vi "Measurement UI.vi"() -> ()   [LabVIEW 2021, in "Gain And Offset_ADC.lvlib"]
uses:
  Gain And Offset_ADC.lvlib
panel:
  in  "MeasGraphs":enum32{"Transfer Function", "Hidden Controls"}(tab)
  out "TransferFunction":cluster{"Waveform":dbl[], "DMM readings":dbl[]}(graph) caption="FreqDomainGraph"
  in  "DMM resource name":string
  out "Offset":dbl
  out "Gain":dbl
  out "Channel name":string
  out "DMM readings":dbl[](array[numeric])
  out "ADC readings":dbl[](array[numeric])
  in  "Digital capture resource name":string
  in  "Analog source resource name":string
  out "MeasTable":string[][](table)
  in  "MeasSettingsOptions":i32(listbox)
  in  "DMM":string="DMM"
  in  "Digital capture":string="Digital capture"
  in  "Analog source":string="Analog source"
  in  "MeasSettings":bool
  in  "ADC parameters":string="ADC parameters"
  in  "DMM resolution":dbl(ring)=7.5 caption="RESOLUTION IN DIGITS" items=["3 1/2"=3.5, "4 1/2"=4.5, "5 1/2"=5.5, "6 1/2"=6.5, "7 1/2"=7.5]
  in  "DMM range":dbl=10.0 caption="RANGE" format="%#_6pV"
  in  "DMMResourceName":refnum<k15> caption="RESOURCE NAME"
  in  "Ramp stop":dbl=4.9 caption="RAMP STOP" format="%#_6pV"
  in  "Ramp start":dbl=-4.9 caption="RAMP START" format="%#_6pV"
  in  "Ramp samples":i32=10 caption="RAMP SAMPLES"
  in  "Analog source sample rate":dbl=1000.0 caption="SAMPLE RATE" format="%#_6pHz"
  in  "Digital capture samples":u32=10000 caption="NUMBER OF SAMPLES"
  in  "Input channel":i32 caption="INPUT CHANNEL" min=0 max=100 step=1
  in  "Full scale range":dbl=10.0 caption="FULL SCALE RANGE" format="%#_6pV"
  in  "Digital capture sample rate":dbl=800000.0 caption="SAMPLE RATE" format="%#_6pS/s"
  in  "DSGResourceName":tag caption="RESOURCE NAME"
  in  "DPIResourceName":refnum<k15> caption="RESOURCE NAME"
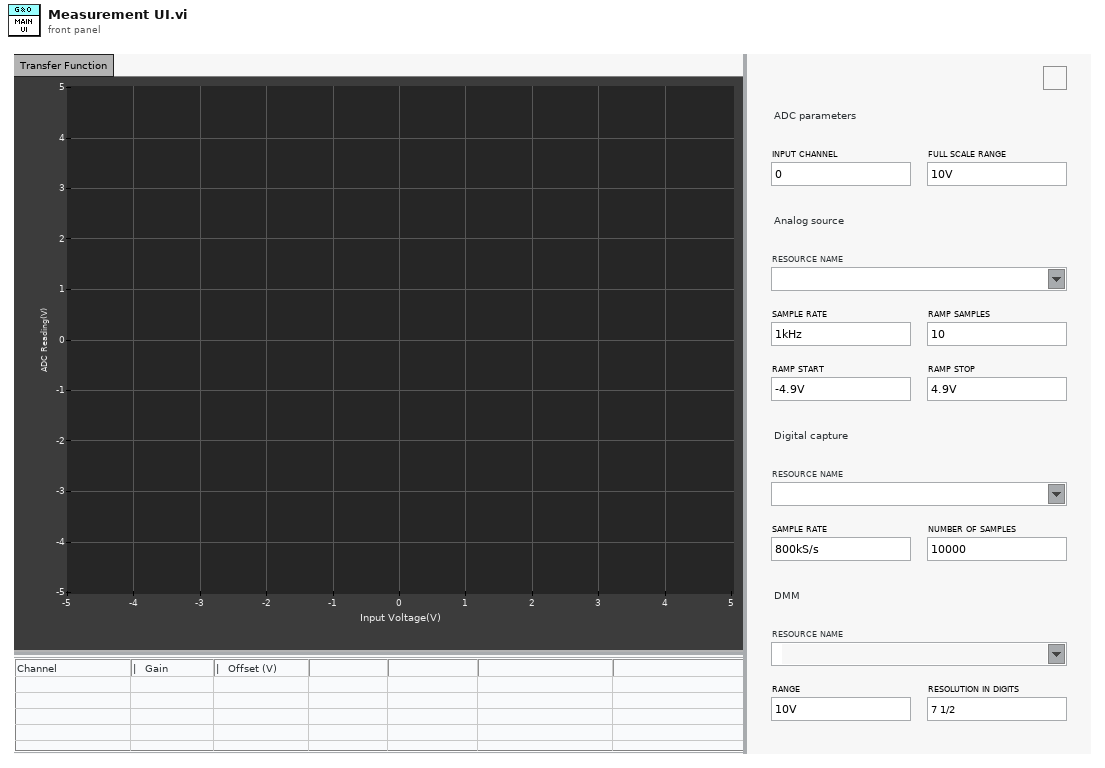
[diagram p1: front panel]
types:
  T1 = enum16{"open", "replace", "create", "open or create", "replace or create", "replace or create with confirmation"}
  T2 = cluster{"ADC readings":dbl[], "DMM readings":dbl[]}
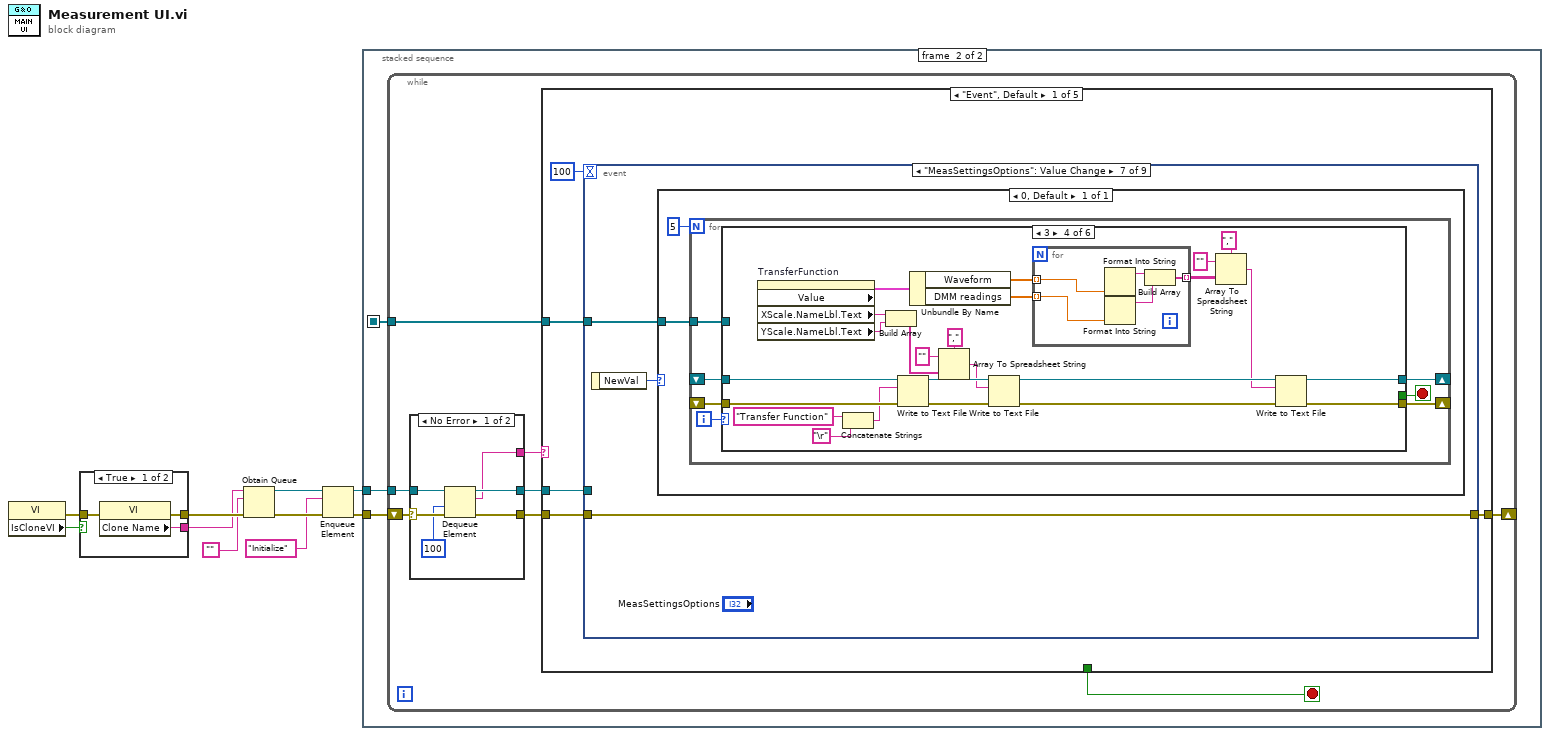
[diagram p0: block diagram]
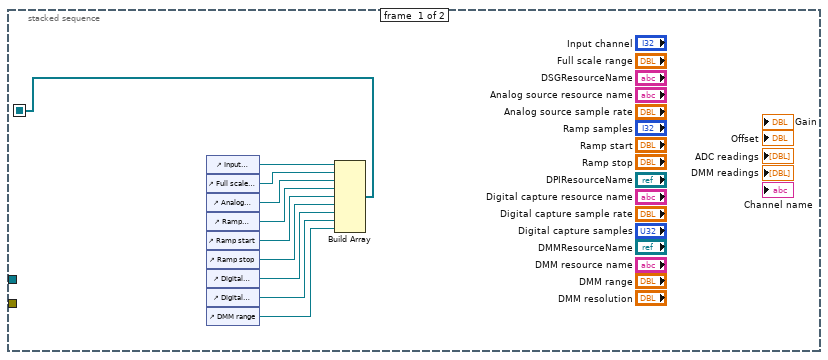
[diagram p2: hidden frame]
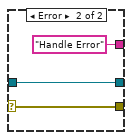
[diagram p3: hidden frame]
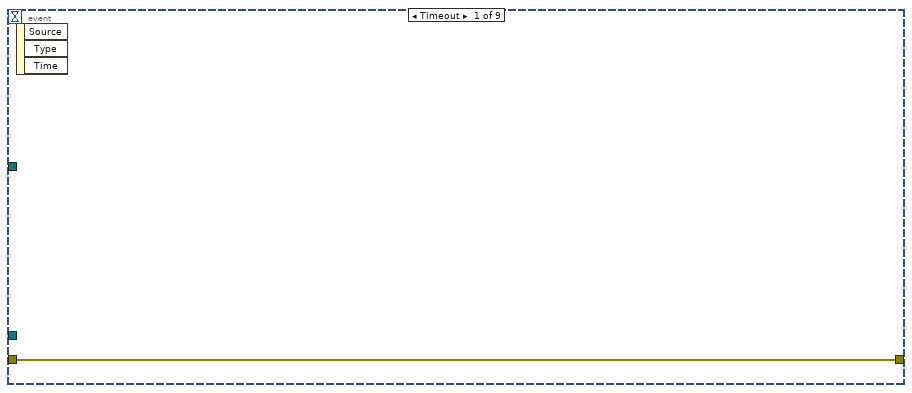
[diagram p4: hidden frame]
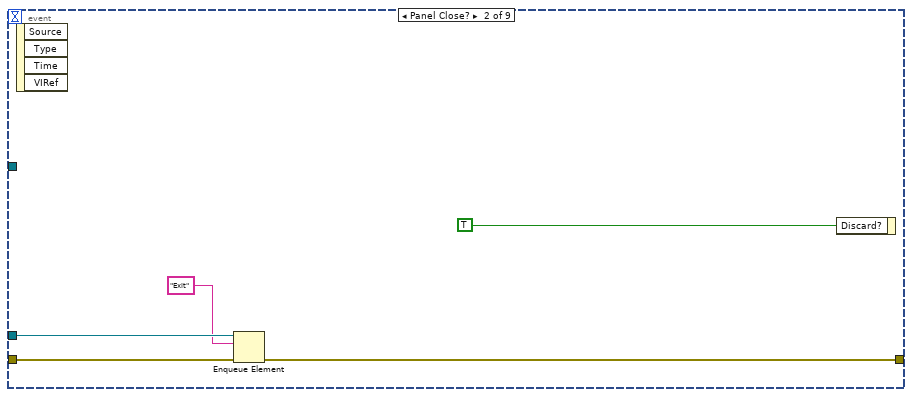
[diagram p5: hidden frame]
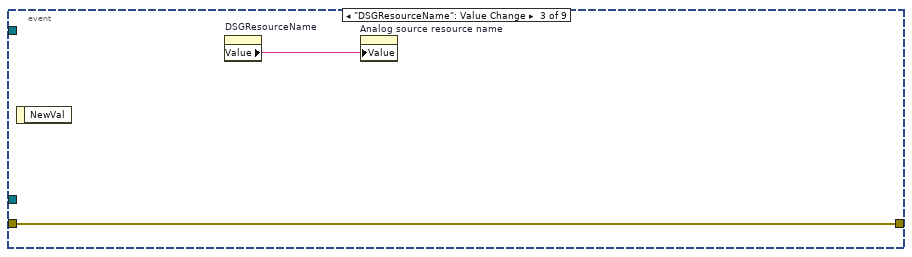
[diagram p6: hidden frame]
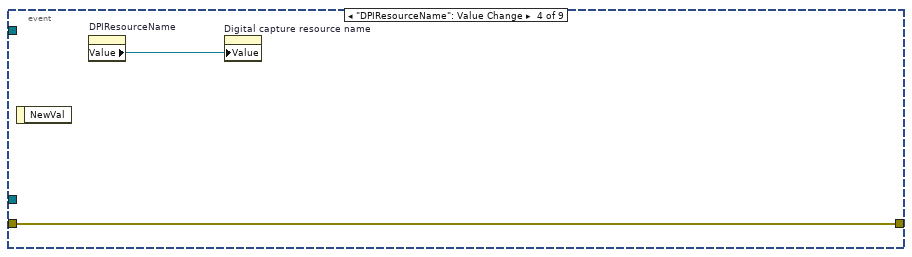
[diagram p7: hidden frame]
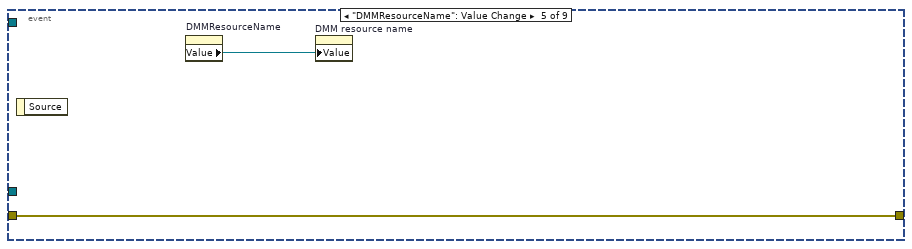
[diagram p8: hidden frame]
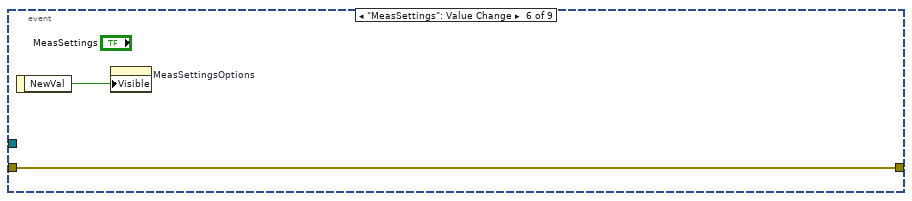
[diagram p9: hidden frame]
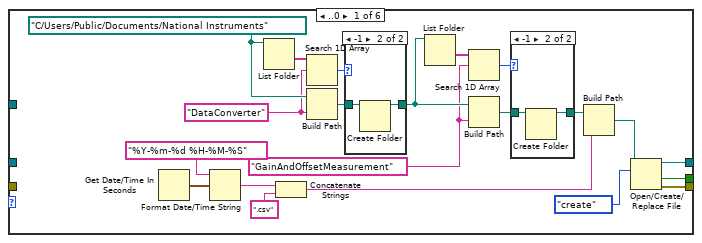
[diagram p10: hidden frame]
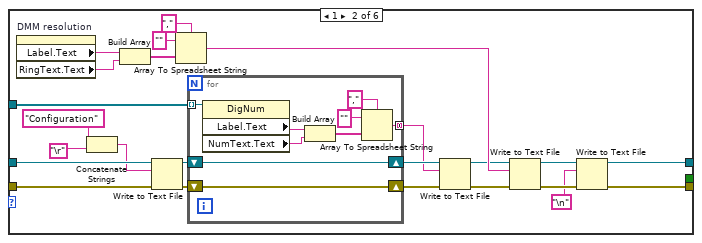
[diagram p13: hidden frame]
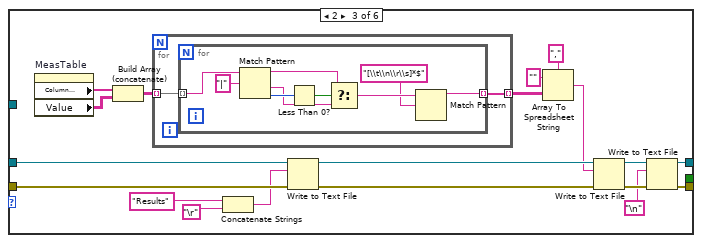
[diagram p14: hidden frame]
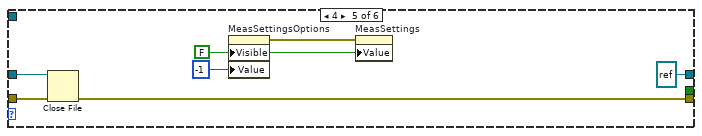
[diagram p15: hidden frame]
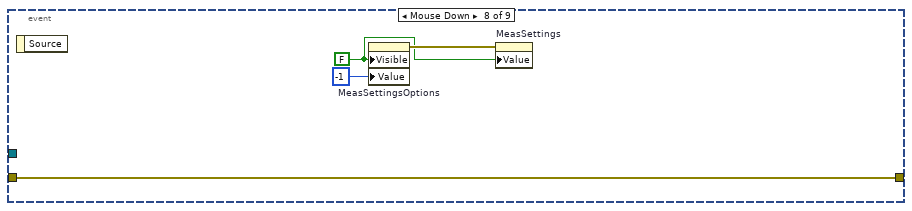
[diagram p17: hidden frame]
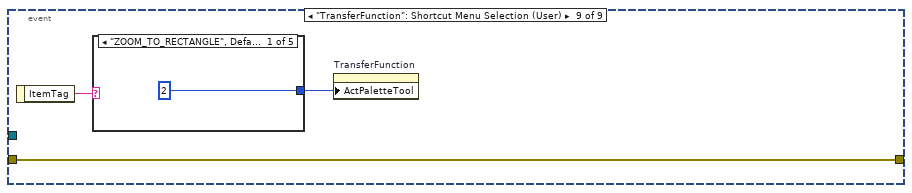
[diagram p18: hidden frame]
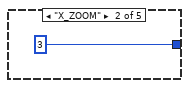
[diagram p19: hidden frame]
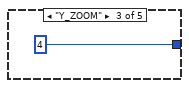
[diagram p20: hidden frame]
diagram:
  n1 = property class="VI"() -> (error out=w1:errorcluster, "IsCloneVI"=w2:bool)  [unwired: 2 in, 1 out]
  n2 = case shown="True" w2 {
    tunnel: [w13 w16] -> w10
    tunnel: [w12 w15] -> w9
    tunnel: w1 -> [w11 w14]
    frame True {
      n3 = property class="VI"(error in=w11) -> (error out=w13:errorcluster, "Clone Name"=w12:string)  [unwired: 1 in, 1 out]
    }
    frame False {
      n4 = property class="VI"(error in=w14) -> (error out=w16:errorcluster, "Name"=w15:string)  [unwired: 1 in, 1 out]
    }
  }
  n5 = Obtain Queue(name (unnamed)=w9, element data type="", error in (no error)=w10) -> (queue out=w6:refnum<queue>, error out=w8:errorcluster)  [unwired: 2 in, 1 out]
  n6 = Enqueue Element(queue=w6, element="Initialize", error in (no error)=w8) -> (queue out=w5:refnum<queue>, error out=w7:errorcluster)  [unwired: 1 in, 1 out]
  n7 = stacked-sequence {
    seq-local: [w17 _] -> [_ w27]
    tunnel: w7 -> [_ w29]
    tunnel: w5 -> [_ w28]
    frame #0 {
      n8 = control-ref of="Input channel"() -> (w26:refnum<vi>)
      n9 = control-ref of="Full scale range"() -> (w25:refnum<vi>)
      n10 = control-ref of="Analog source sample rate"() -> (w24:refnum<vi>)
      n11 = control-ref of="Ramp samples"() -> (w23:refnum<vi>)
      n12 = control-ref of="Ramp start"() -> (w22:refnum<vi>)
      n13 = control-ref of="Ramp stop"() -> (w21:refnum<vi>)
      n14 = control-ref of="Digital capture sample rate"() -> (w20:refnum<vi>)
      n15 = control-ref of="Digital capture samples"() -> (w19:refnum<vi>)
      n16 = control-ref of="DMM range"() -> (w18:refnum<vi>)
      n17 = Build Array(w26, w25, w24, w23, w22, w21, w20, w19, w18) -> (w17:refnum<vi>[])
    }
    frame #1 {
      n18 = while {
        shift-right: [w32] -> _
        shift-left: w29 -> [w37]
        tunnel: w28 -> [w35]
        tunnel: w27 -> [w30]
        stop <- w31 stop-if-true
        n19 = case shown="No Error" w37 {
          selector: w37 -> [w43 w46]
          tunnel: [w42 w46] -> w36
          tunnel: w35 -> [w41 w45]
          tunnel: [w40 w45] -> w34
          tunnel: [w39 "Handle Error"] -> w33
          frame No Error {
            n20 = Dequeue Element(queue=w41, timeout in ms (-1)=100, error in (no error)=w43) -> (queue out=w40:refnum<queue>, element=w39:string, error out=w42:errorcluster)  [unwired: 1 out]
          }
          frame Error {
          }
        }
        n21 = case shown="\"Event\", Default" w33 {
          tunnel: w36 -> [w50 w225 w239 w249 w250]
          tunnel: w34 -> [w48 _ _ w247 _]
          tunnel: [w51 w225 w239 w244 w250] -> w32
          tunnel: [_ FALSE _ TRUE _] -> w31
          tunnel: w30 -> [w47 _ _ _ _]
          frame "Event", Default {
            n22 = event shown="[6] \"MeasSettingsOptions\": Value Change" {
              selector: _ -> [_ _ _ _ _ _ _ _ _]
              dyn-events: _ -> [_ _ _ _ _ _ _ _ _]
              timeout: 100 -> [_ _ _ _ _ _ _ _ _]
              tunnel: [w52 w55 w59 w60 w62 w65 w68 w209 w210] -> w51
              tunnel: w50 -> [w52 w56 w59 w60 w62 w65 w68 w209 w210]
              tunnel: w48 -> [_ w54 _ _ _ _ _ _ _]
              tunnel: w47 -> [_ _ _ _ _ _ w66 _ _]
              event Timeout {
                n23 = event-data() -> ()  [unwired: 1 in, 3 out]
              }
              event Panel Close? {
                n24 = event-data() -> ()  [unwired: 1 in, 4 out]
                n25 = Enqueue Element(queue=w54, element="Exit", error in (no error)=w56) -> (error out=w55:errorcluster)  [unwired: 1 in, 2 out]
                n26 = event-data("Discard?"=TRUE) -> ()  [unwired: 1 in, 1 out]
              }
              event "DSGResourceName": Value Change {
                n27 = event-data() -> ()  [unwired: 1 in, 1 out]
                n28 = property on="DSGResourceName" class="DAQmxName"() -> ("Value"=w58:string)  [unwired: 2 in, 2 out]
                n29 = property on="Analog source resource name" class="Str"("Value"=w58) -> ()  [unwired: 2 in, 2 out]
              }
              event "DPIResourceName": Value Change {
                n30 = event-data() -> ()  [unwired: 1 in, 1 out]
                n31 = property on="DPIResourceName" class="IVIName"() -> ("Value"=w61:refnum<k15>)  [unwired: 2 in, 2 out]
                n32 = property on="Digital capture resource name" class="Str"("Value"=w61) -> ()  [unwired: 2 in, 2 out]
              }
              event "DMMResourceName": Value Change {
                n33 = event-data() -> ()  [unwired: 1 in, 1 out]
                n34 = property on="DMMResourceName" class="IVIName"() -> ("Value"=w63:refnum<k15>)  [unwired: 2 in, 2 out]
                n35 = property on="DMM resource name" class="Str"("Value"=w63) -> ()  [unwired: 2 in, 2 out]
              }
              event "MeasSettings": Value Change {
                n36 = event-data() -> ("NewVal"=w64:bool)  [unwired: 1 in]
                n37 = property on="MeasSettingsOptions" class="LstBox (strict)"("Visible"=w64) -> ()  [unwired: 2 in, 2 out]
              }
              event "MeasSettingsOptions": Value Change {
                n38 = event-data() -> ("NewVal"=w67:i32)  [unwired: 1 in]
                n39 = case shown="0, Default" w67 {
                  tunnel: w66 -> [w69]
                  frame 0, Default {
                    n40 = for {
                      N: 5 -> [_]
                      shift-right: [w75] -> _
                      shift-left: _ -> [w74]
                      shift-right: [w73] -> _
                      shift-left: _ -> [w72]
                      tunnel: w69 -> [w71]
                      i -> [w77]
                      stop <- w76 stop-if-true
                      n41 = case shown="3" w77 {
                        tunnel: [w91 _ _ _ _ _] -> w76
                        tunnel: [w97 w108 w143 w177 refnum<file> refnum ("refnum out") w205] -> w75
                        tunnel: w74 -> [_ w126 w156 w191 w200 w205]
                        tunnel: [w90 w106 w142 w176 w198 w204] -> w73
                        tunnel: w72 -> [_ w124 w155 w190 w199 w204]
                        tunnel: w71 -> [_ w128 _ _ _ _]
                        frame ..0 {
                          w86 = "GainAndOffsetMeasurement" ("prompt")
                          w93 = "DataConverter" ("prompt")
                          w96 = path "C:/Users/Public/Documents/National Instruments" ("base path")
                          n42 = Get Date/Time In Seconds() -> (seconds since 1Jan1904=w83:timestamp)
                          n43 = Format Date/Time String(time format string (%c)="%Y-%m-%d %H-%M-%S", seconds (now)=w83) -> (date/time string=w82:string)  [unwired: 1 in]
                          n44 = List Folder(path=w96) -> (folder names=w94:string[])  [unwired: 3 in, 3 out]
                          n45 = Concatenate Strings(w82, ".csv" ("string")) -> (w79:string)
                          n46 = Search 1D Array(1D array=w94, element=w93) -> (index of element=w92:i32)  [unwired: 1 in]
                          n47 = Build Path(base path=w96, name or relative path=w93) -> (appended path=w95:path)
                          n48 = case shown="-1" w92 {
                            tunnel: w95 -> [w102 w104]
                            tunnel: [w102 w103] -> w87
                            frame Default {
                            }
                            frame -1 {
                              n49 = Create Folder(path (use dialog)=w104) -> (created path=w103:path)  [unwired: 2 in, 2 out]
                            }
                          }
                          n50 = List Folder(path=w87) -> (folder names=w89:string[])  [unwired: 3 in, 3 out]
                          n51 = Search 1D Array(1D array=w89, element=w86) -> (index of element=w88:i32)  [unwired: 1 in]
                          n52 = Build Path(base path=w87, name or relative path=w86) -> (appended path=w85:path)
                          n53 = case shown="-1" w88 {
                            tunnel: w85 -> [w99 w101]
                            tunnel: [w99 w100] -> w80
                            frame Default {
                            }
                            frame -1 {
                              n54 = Create Folder(path (use dialog)=w101) -> (created path=w100:path)  [unwired: 2 in, 2 out]
                            }
                          }
                          n55 = Build Path(base path=w80, name or relative path=w79) -> (appended path=w78:path)
                          n56 = Open/Create/Replace File(file path (use dialog)=w78, operation (0:open)=T1."create") -> (refnum out=w97:refnum<file>, cancelled=w91:bool, error out=w90:errorcluster)  [unwired: 4 in]
                        }
                        frame 1 {
                          n57 = property on="DMM resolution" class="Ring (strict)"() -> ("Label.Text"=w120:string, "RingText.Text"=w119:string)  [unwired: 2 in, 2 out]
                          n58 = Concatenate Strings("Configuration" ("format string"), "\r") -> (w121:string)
                          n59 = Build Array(w120, w119) -> (w116:string[])
                          n60 = Write to Text File(file (use dialog)=w126, text=w121, error in=w124) -> (refnum out=w127:refnum<file>, error out=w125:errorcluster)  [unwired: 1 in, 1 out]
                          n61 = Array To Spreadsheet String(delimiter (Tab)=",", array=w116, 3:"" ("format string")) -> (spreadsheet string=w115:string)
                          n62 = for {
                            tunnel: w128 -> [w137] mode=indexing
                            shift-right: [w134] -> w114
                            shift-left: w127 -> [w134]
                            shift-right: [w133] -> w112
                            shift-left: w125 -> [w133]
                            tunnel: [w129] -> w110 mode=concatenating
                            n63 = property class="DigNum"(reference=w137) -> ("Label.Text"=w136:string, "NumText.Text"=w135:string)  [unwired: 1 in, 2 out]
                            n64 = Build Array(w136, w135) -> (w130:string[])
                            n65 = Array To Spreadsheet String(delimiter (Tab)=",", array=w130, 3:"" ("format string")) -> (spreadsheet string=w129:string)
                          }
                          n66 = Write to Text File(file (use dialog)=w114, text=w110, error in=w112) -> (refnum out=w113:refnum<file>, error out=w111:errorcluster)  [unwired: 1 in, 1 out]
                          n67 = Write to Text File(file (use dialog)=w113, text=w115, error in=w111) -> (refnum out=w109:refnum<file>, error out=w107:errorcluster)  [unwired: 1 in, 1 out]
                          n68 = Write to Text File(file (use dialog)=w109, text="\n", error in=w107) -> (refnum out=w108:refnum<file>, error out=w106:errorcluster)  [unwired: 1 in, 1 out]
                        }
                        frame 2 {
                          n69 = property on="MeasTable" class="Tbl (strict)"() -> ("Column Headers[]"=w153:string[], "Value"=w152:string[][])  [unwired: 2 in, 2 out]
                          n70 = Build Array (concatenate)(w153, w152) -> (w151:string[][])
                          n71 = for {
                            tunnel: w151 -> [w158] mode=indexing
                            tunnel: [w157] -> w150 mode=indexing
                            n72 = for {
                              tunnel: w158 -> [w160] mode=indexing
                              tunnel: [w159] -> w157 mode=indexing
                              n73 = Match Pattern(string=w160, regular expression="|") -> (before substring=w164:string, after substring=w163:string, offset past match=w166:i32)  [unwired: 1 in, 1 out]
                              n74 = Less Than 0?(x=w166) -> (x < 0?=w165:bool)
                              n75 = Select(t=w164, s=w165, f=w163) -> (s? t:f=w162:string)
                              n76 = Match Pattern(string=w162, regular expression="[\\t\\n\\r\\s]*$") -> (before substring=w159:string)  [unwired: 1 in, 3 out]
                            }
                          }
                          n77 = Concatenate Strings("Results" ("element"), "\r") -> (w138:string)
                          n78 = Write to Text File(file (use dialog)=w156, text=w138, error in=w155) -> (refnum out=w154:refnum<file>, error out=w146:errorcluster)  [unwired: 1 in, 1 out]
                          n79 = Array To Spreadsheet String(delimiter (Tab)=",", array=w150, 3:"" ("format string")) -> (spreadsheet string=w147:string)
                          n80 = Write to Text File(file (use dialog)=w154, text=w147, error in=w146) -> (refnum out=w145:refnum<file>, error out=w144:errorcluster)  [unwired: 1 in, 1 out]
                          n81 = Write to Text File(file (use dialog)=w145, text="\n", error in=w144) -> (refnum out=w143:refnum<file>, error out=w142:errorcluster)  [unwired: 1 in, 1 out]
                        }
                        frame 3 {
                          n82 = property on="TransferFunction" class="XYGraph (strict)"() -> ("Value"=w170:cluster{"Waveform":dbl[], "DMM readings":dbl[]}, "XScale.NameLbl.Text"=w187:string, "YScale.NameLbl.Text"=w186:string)  [unwired: 2 in, 2 out]
                          n83 = Concatenate Strings("Transfer Function" ("string"), "\r") -> (w188:string)
                          n84 = Build Array(w187, w186) -> (w185:string[])
                          n85 = Write to Text File(file (use dialog)=w191, text=w188, error in=w190) -> (refnum out=w182:refnum<file>, error out=w181:errorcluster)  [unwired: 1 in, 1 out]
                          n86 = Unbundle By Name(w170) -> ("Waveform"=w171:dbl[], "DMM readings"=w172:dbl[])
                          n87 = Array To Spreadsheet String(delimiter (Tab)=",", array=w185, 3:"" ("format string")) -> (spreadsheet string=w180:string)
                          n88 = Write to Text File(file (use dialog)=w182, text=w180, error in=w181) -> (refnum out=w179:refnum<file>, error out=w178:errorcluster)  [unwired: 1 in, 1 out]
                          n89 = for {
                            tunnel: w171 -> [w193] mode=indexing
                            tunnel: w172 -> [w192] mode=indexing
                            tunnel: [w194] -> w173 mode=indexing
                            n90 = Format Into String(w193) -> (resulting string=w195:string)  [unwired: 3 in, 1 out]
                            n91 = Format Into String(w192) -> (resulting string=w196:string)  [unwired: 3 in, 1 out]
                            n92 = Build Array(w195, w196) -> (w194:string[])
                          }
                          n93 = Array To Spreadsheet String(delimiter (Tab)=",", array=w173, 3:"" ("format string")) -> (spreadsheet string=w169:string)
                          n94 = Write to Text File(file (use dialog)=w179, text=w169, error in=w178) -> (refnum out=w177:refnum<file>, error out=w176:errorcluster)  [unwired: 1 in, 1 out]
                        }
                        frame 4 {
                          w202 = FALSE ("Visible")
                          n95 = Close File(refnum=w200, error in=w199) -> (error out=w198:errorcluster)  [unwired: 1 out]
                          n96 = property on="MeasSettingsOptions" class="LstBox (strict)"("Visible"=w202, "Value"=-1 ("MeasSettingsOptions")) -> (error out=w203:errorcluster)  [unwired: 2 in, 1 out]
                          n97 = property on="MeasSettings" class="Bool (strict)"(error in=w203, "Value"=w202) -> ()  [unwired: 1 in, 2 out]
                        }
                        frame Default {
                        }
                      }
                    }
                  }
                }
              }
              event Mouse Down {
                w207 = FALSE ("Visible")
                n98 = event-data() -> ()  [unwired: 1 in, 1 out]
                n99 = property on="MeasSettingsOptions" class="LstBox (strict)"("Visible"=w207, "Value"=-1 ("MeasSettingsOptions")) -> (error out=w208:errorcluster)  [unwired: 2 in, 1 out]
                n100 = property on="MeasSettings" class="Bool (strict)"(error in=w208, "Value"=w207) -> ()  [unwired: 1 in, 2 out]
              }
              event "TransferFunction": Shortcut Menu Selection (User) {
                n101 = event-data() -> ("ItemTag"=w212:string)  [unwired: 1 in]
                n102 = case shown="\"ZOOM_TO_RECTANGLE\", Default" w212 {
                  tunnel: [2 ("Palette:Active Tool") 3 ("Palette:Active Tool") 4 ("Palette:Active Tool") 5 ("Palette:Active Tool") 1 ("Palette:Active Tool")] -> w211
                  frame "ZOOM_TO_RECTANGLE", Default {
                  }
                  frame "X_ZOOM" {
                  }
                  frame "Y_ZOOM" {
                  }
                  frame "ZOOM_TO_FIT" {
                  }
                  frame "PANNING_TOOL" {
                  }
                }
                n103 = property on="TransferFunction" class="XYGraph (strict)"("ActPaletteTool"=w211) -> ()  [unwired: 2 in, 2 out]
              }
            }
          }
          frame "Initialize" {
            w222 = string[] ["Export data"] ("Item Names")
            w223 = "<Select Device>"
            n104 = property on="DSGResourceName" class="DAQmxName"("Value"=w223) -> ()  [unwired: 2 in, 2 out]
            n105 = property on="DPIResourceName" class="IVIName"("Value"=w223) -> ()  [unwired: 2 in, 2 out]
            n106 = property on="DMMResourceName" class="IVIName"("Value"=w223) -> ()  [unwired: 2 in, 2 out]
            n107 = property on="MeasSettingsOptions" class="LstBox (strict)"("Item Names"=w222, "Value"=-1 ("MeasSettingsOptions"), "Visible"=FALSE, "Disabled Items"=i32[] []) -> ()  [unwired: 2 in, 2 out]
            n108 = property on="TransferFunction" class="XYGraph (strict)"("ActPaletteTool"=2 ("Palette:Active Tool")) -> ()  [unwired: 2 in, 2 out]
            n109 = for {
              tunnel: w222 -> [_] mode=indexing
              i -> [w227]
              n110 = property on="MeasSettingsOptions" class="LstBox (strict)"("Active Row"=w227, "Cell Height"=30 ("Active Row:Cell Height")) -> ()  [unwired: 2 in, 2 out]
            }
          }
          frame "Post UI Update" {
            # "This case will be triggered, after framework updates the User interface with result values."
            n111 = local read "Offset"() -> (w237:dbl)
            n112 = local read "DMM readings"() -> (w229:dbl[])
            n113 = local read "Gain"() -> (w238:dbl)
            n114 = local read "ADC readings"() -> (w230:dbl[])
            n115 = Build Array(w238, w237) -> (w236:dbl[])
            n116 = Bundle("ADC readings"=w230, "DMM readings"=w229) -> (→"TransferFunction":T2)  [unwired: 1 in]
            n117 = local read "Channel name"() -> (w231:string)
            n118 = for {
              tunnel: w236 -> [w240] mode=indexing
              tunnel: "|   " ("initial string") -> [w241]
              tunnel: [w242] -> w234 mode=indexing
              n119 = Format Into String(initial string=w241, w240) -> (resulting string=w242:string)  [unwired: 2 in, 1 out]
            }
            n120 = Build Array (concatenate)(w231, w234) -> (w233:string[])
            n121 = Build Array(w233) -> (→"MeasTable":string[][])
          }
          frame "Exit" {
            # "This case is triggered to close the User Interface from framework"
            n122 = Flush Queue(queue=w247, error in (no error)=w249) -> (queue out=w246:refnum<queue>, error out=w245:errorcluster)  [unwired: 1 out]
            n123 = Release Queue(queue=w246, force destroy? (F)=TRUE, error in (no error)=w245) -> (error out=w244:errorcluster)  [unwired: 2 out]
          }
          frame "Handle Error" {
          }
        }
      }
    }
  }
